vi "ConsumeACKs(byID).vi"(8 "error in (no error)":errorcluster, 10 "Packet Identifier":u16 format="%016b", 11 "Session in":refnum<class "Session.lvclass">) -> (0 "error out":errorcluster, 3 "Session out":refnum<class "Session.lvclass">)   [LabVIEW 2013, in "MQTT Server.lvlib" / "Session.lvclass"]
uses:
  Session.lvclass
  Session.lvclass/Session.ctl
  Control Packets/ControlPacket/ControlPacket.lvclass
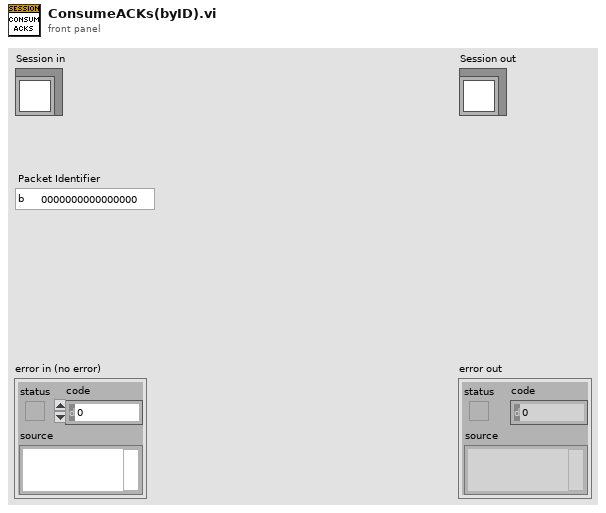
[diagram p1: front panel]
types:
  T1 = typedef "MQTT Server.lvlib/Session.lvclass/Session State -- cluster.ctl" = cluster{"CleanSession":bool, "Client ID":string, "Subscriptions":T2[], "Pending Transmissions":T4[], "Pending ACKs":T5[]}
  T2 = typedef "SUBSCRIBE.lvclass/Topic Subscription -- cluster.ctl" = cluster{"Topic Filter":string, "QoS":T3}
  T3 = typedef "ControlPacket.lvclass/QualityOfService -- enum.ctl" = enum16{"0 (At Most Once)", "1 (At Least Once)", "2 (Exactly Once)"}
  T4 = typedef "ControlPacket.lvclass/Pending Transmission -- cluster.ctl" = cluster{"Message":refnum<class "ControlPacket.lvclass">, "QoS":T3, "Tx-Rx":bool}
  T5 = typedef "MQTT Server.lvlib/Session.lvclass/Pending ACKs -- cluster.ctl" = cluster{"Message":refnum<class "ControlPacket.lvclass">, "[ACK]":refnum<notifier>[], "Packet Identifier":u16}
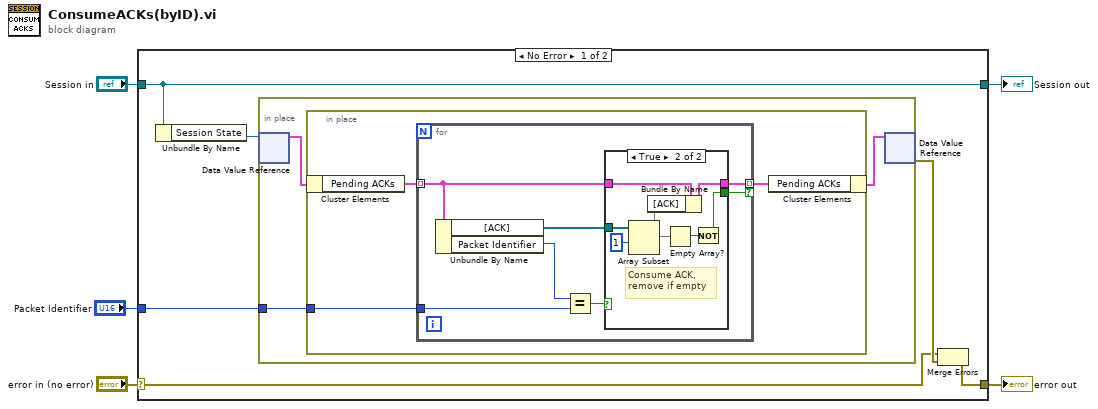
[diagram p0: block diagram]
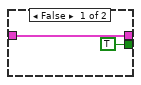
[diagram p2: hidden frame]
diagram:
  n1 = case shown="No Error" "error in (no error)" {
    selector: "error in (no error)" -> [w7 w34]
    tunnel: [w6 w34] -> w2
    tunnel: [w11 w35] -> w1
    tunnel: "Session in" -> [w11 w35]
    tunnel: "Packet Identifier" -> [w9 _]
    frame No Error {
      n2 = Unbundle By Name(w11) -> ("Session State"=w10:refnum<data-value>)
      n3 = in-place {
        in-place-border: w9 -> [w12]
        n4 = in-place-dvr #1(w10) -> (w14:T1)  [unwired: 1 out]
        n5 = in-place {
          in-place-border: w12 -> [w16]
          n6 = in-place-cluster #2(w14) -> ("Pending ACKs"=w15:T5[])
          n7 = for {
            tunnel: w15 -> [w19] mode=indexing
            tunnel: [w20] -> w17 mode=indexing if=w24
            tunnel: w16 -> [w22]
            n8 = Unbundle By Name(w19) -> ("[ACK]"=w18:refnum<notifier>[], "Packet Identifier"=w23:u16)
            n9 = Equal?(x=w23, y=w22) -> (x = y?=w21:bool)
            n10 = case shown="True" w21 {
              tunnel: [TRUE w27] -> w24
              tunnel: [w25 w30] -> w20
              tunnel: w19 -> [w25 w31]
              tunnel: w18 -> [_ w33]
              frame False {
              }
              frame True {
                # "Consume ACK,\nremove if empty"
                n11 = Array Subset(array=w33, index=1) -> (w29:refnum<notifier>[])  [unwired: 1 in]
                n12 = Bundle By Name(cluster=w31, "[ACK]"=w29) -> (w30:T5)
                n13 = Empty Array?(array=w29) -> (empty?=w28:bool)
                n14 = Not(x=w28) -> (.not. x?=w27:bool)
              }
            }
          }
          n15 = in-place-cluster #2("Pending ACKs"=w17) -> (w13:T1)
        }
        n16 = in-place-dvr #1(w13) -> (w8:errorcluster)  [unwired: 1 out]
      }
      n17 = Merge Errors(w7, w8) -> (w6:errorcluster)
    }
    frame Error {
    }
  }
  "error out" <- w2
  "Session out" <- w1
